vi "Define CellStyle.vi"(8 "error in (no error)":errorcluster, 10 "CellStyle":T1 {"Alignment" items=["NotSet"=0, "TopLeft"=1, "TopCenter"=2, "TopRight"=4, "MiddleLeft"=16, "MiddleCenter"=32, "MiddleRight"=64, "BottomLeft"=256, "BottomCenter"=512, "BottomRight"=1024]; "WrapMode" items=["NotSet", "True", "False"]}) -> (0 "error out":errorcluster, 3 "CellStyle out":refnum<class "CellStyle.lvclass">)   [LabVIEW 2016, in "DataGrid.lvlib" / "CellStyle.lvclass"]
uses:
  <userlib>/LabVIEWdotNetDataGrid/source/CellStyle/CellStyle.lvclass
  <userlib>/LabVIEWdotNetDataGrid/source/CellStyle/CellStyleCluster.ctl
  <userlib>/LabVIEWdotNetDataGrid/source/Color/Color.lvclass
  <userlib>/LabVIEWdotNetDataGrid/source/Font/Font.lvclass
  <userlib>/LabVIEWdotNetDataGrid/source/Font/Font.lvclass/Font.ctl
  System.Windows.Forms
  <userlib>/LabVIEWdotNetDataGrid/source/CellStyle/CellStyle.lvclass/CellStyle.ctl
  <userlib>/LabVIEWdotNetDataGrid/source/Font/Properties/Read Font.vi
  System.Drawing
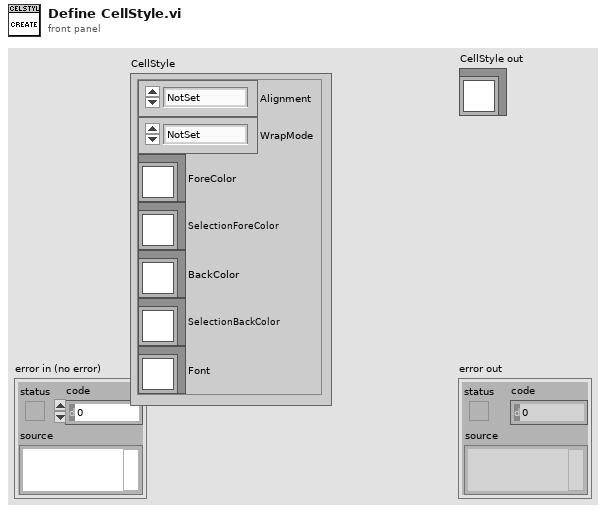
[diagram p1: front panel]
types:
  T1 = typedef "DataGrid.lvlib/CellStyle.lvclass/CellStyleCluster.ctl" = cluster{"Alignment":i32, "WrapMode":i32, "ForeColor":refnum<class "Color.lvclass">, "SelectionForeColor":refnum<class "Color.lvclass">, "BackColor":refnum<class "Color.lvclass">, "SelectionBackColor":refnum<class "Color.lvclass">, "Font":refnum<class "Font.lvclass">}
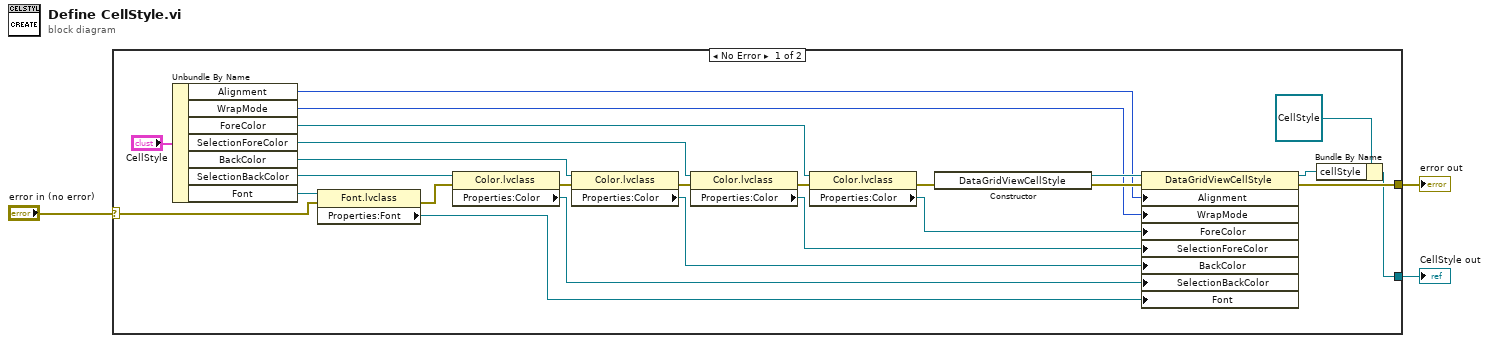
[diagram p0: block diagram]
diagram:
  n1 = case shown="No Error" "error in (no error)" {
    selector: "error in (no error)" -> [w11 w29]
    tunnel: [w27 w29] -> w2
    tunnel: [w13 _] -> w1
    frame No Error {
      n2 = Unbundle By Name("CellStyle") -> ("Alignment"=w5:i32, "WrapMode"=w4:i32, "ForeColor"=w25:refnum<class "Color.lvclass">, "SelectionForeColor"=w23:refnum<class "Color.lvclass">, "BackColor"=w22:refnum<class "Color.lvclass">, "SelectionBackColor"=w21:refnum<class "Color.lvclass">, "Font"=w12:refnum<class "Font.lvclass">)
      n3 = property class="Font.lvclass"(reference=w12, error in=w11) -> (error out=w9:errorcluster, "Properties:Font"=w10:refnum<k24>)  [unwired: 1 out]
      n4 = property class="Color.lvclass"(reference=w21, error in=w9) -> (error out=w17:errorcluster, "Properties:Color"=w18:refnum<k24>)  [unwired: 1 out]
      n5 = property class="Color.lvclass"(reference=w22, error in=w17) -> (error out=w16:errorcluster, "Properties:Color"=w19:refnum<k24>)  [unwired: 1 out]
      n6 = property class="Color.lvclass"(reference=w23, error in=w16) -> (error out=w15:errorcluster, "Properties:Color"=w20:refnum<k24>)  [unwired: 1 out]
      n7 = property class="Color.lvclass"(reference=w25, error in=w15) -> (error out=w6:errorcluster, "Properties:Color"=w24:refnum<k24>)  [unwired: 1 out]
      n8 = constructor class="DataGridViewCellStyle"(error in=w6) -> (reference out=w8:refnum<k24>, error out=w7:errorcluster)  [unwired: 2 in, 1 out]
      n9 = property class="DataGridViewCellStyle"(reference=w8, error in=w7, "Alignment"=w5, "WrapMode"=w4, "ForeColor"=w24, "SelectionForeColor"=w20, "BackColor"=w19, "SelectionBackColor"=w18, "Font"=w10) -> (reference out=w28:refnum<k24>, error out=w27:errorcluster)
      n10 = Bundle By Name(cluster=refnum<class "CellStyle.lvclass"> refnum ("CellStyle in"), "cellStyle"=w28) -> (w13:refnum<class "CellStyle.lvclass">)
    }
    frame Error {
    }
  }
  "error out" <- w2
  "CellStyle out" <- w1
